vi "Read Name.vi"(8 "error in (no error)":errorcluster, 11 "Subscription":refnum<class "Subscription.lvclass">) -> (0 "error out":errorcluster, 2 "Name":string, 3 "Subscription out":refnum<class "Subscription.lvclass">)   [LabVIEW 2015, in "NI_AWS_SNS.lvlib" / "Subscription.lvclass"]
uses:
  Subscription.lvclass
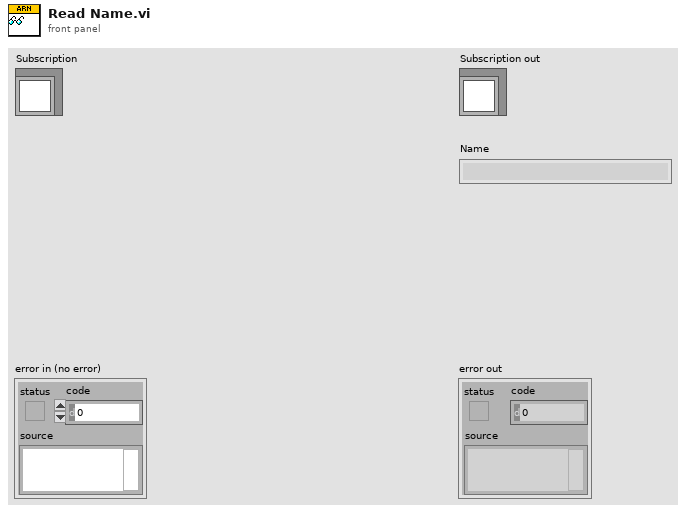
[diagram p1: front panel]
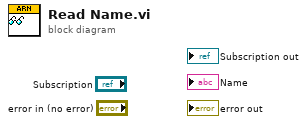
[diagram p0: block diagram]
diagram:
